vi "Set Timing Source.vi"(8 "error in (no error)":errorcluster, 10 "Timing Source":enum16{"Automatic", "Custom Device"}(ring), 11 "Item Ref in":T1 format="%.0x") -> (0 "error out":errorcluster, 3 "Item Ref out":T1 format="%.0x")   [LabVIEW 2016, in "Scan Engine Custom Device.lvlib"]
uses:
  Scan Engine Custom Device.lvlib
  <vilib>/NI Veristand/Custom Device Tools/Custom Device Utility Library/Custom Device Utility Library.lvlib
  <vilib>/NI Veristand/Custom Device API/Custom Device API.lvlib
  NationalInstruments.VeriStand.SystemStorage
  <vilib>/NI Veristand/Custom Device API/Custom Device Item Ref.ctl
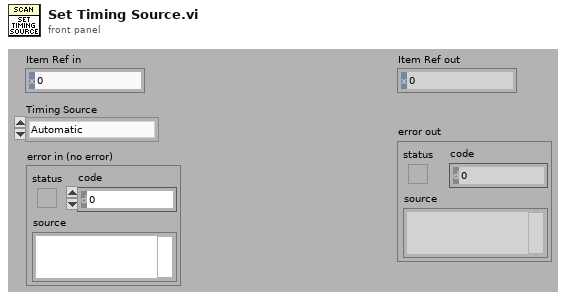
[diagram p1: front panel]
types:
  T1 = typedef "Custom Device API.lvlib/Custom Device Item Ref.ctl" = u64
  T2 = typedef "Custom Device API.lvlib/Custom Device Pointer.ctl" = refnum<k24>
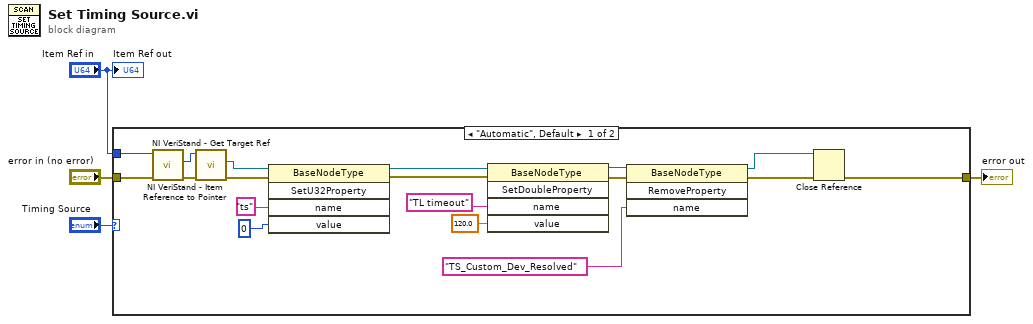
[diagram p0: block diagram]
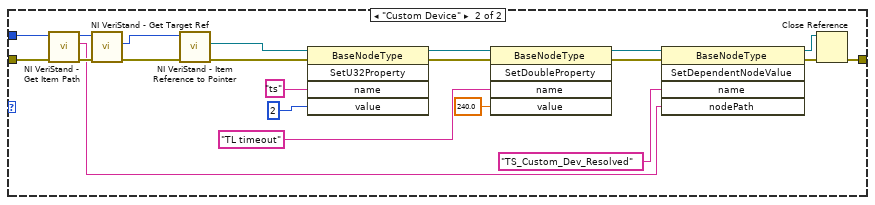
[diagram p2: hidden frame]
diagram:
  n1 = case shown="\"Automatic\", Default" "Timing Source" {
    tunnel: "Item Ref in" -> [w21 w43]
    tunnel: "error in (no error)" -> [w22 w42]
    tunnel: [w11 w29] -> w2
    frame "Automatic", Default {
      n2 = call <vilib>:"NI VeriStand - Get Target Ref.vi"("error in"=w22, "Item Ref in"=w21) -> ("error out"=w20:errorcluster, "Target Ref"=w19:T1)  [unwired: 6 in, 2 out]
      n3 = call <vilib>:"NI VeriStand - Item Reference to Pointer.vi"("error in (no error)"=w20, "Item Ref in"=w19) -> ("error out"=w18:errorcluster, "Node Pointer"=w17:T2)  [unwired: 6 in, 2 out]
      n4 = invoke class="BaseNodeType" method="SetU32Property"(reference=w17, error in=w18, "name"="ts", "value"=u32 0) -> (reference out=w9:T2, error out=w6:errorcluster)  [unwired: 1 in, 3 out]
      n5 = invoke class="BaseNodeType" method="SetDoubleProperty"(reference=w9, error in=w6, "name"="TL timeout", "value"=120.0) -> (reference out=w8:T2, error out=w7:errorcluster)  [unwired: 1 in, 3 out]
      n6 = invoke class="BaseNodeType" method="RemoveProperty"(reference=w8, error in=w7, "name"="TS_Custom_Dev_Resolved") -> (reference out=w13:T2, error out=w12:errorcluster)  [unwired: 1 in, 2 out]
      n7 = Close Reference(reference=w13, error in (no error)=w12) -> (error out=w11:errorcluster)
    }
    frame "Custom Device" {
      n8 = call <vilib>:"NI VeriStand - Get Item Path.vi"("error in (no error)"=w42, "Item Ref in"=w43) -> ("error out"=w41:errorcluster, "Path"=w33:string, "Item Ref out"=w40:T1)  [unwired: 6 in, 1 out]
      n9 = call <vilib>:"NI VeriStand - Get Target Ref.vi"("error in"=w41, "Item Ref in"=w40) -> ("error out"=w39:errorcluster, "Target Ref"=w38:T1)  [unwired: 6 in, 2 out]
      n10 = call <vilib>:"NI VeriStand - Item Reference to Pointer.vi"("error in (no error)"=w39, "Item Ref in"=w38) -> ("error out"=w34:errorcluster, "Node Pointer"=w37:T2)  [unwired: 6 in, 2 out]
      n11 = invoke class="BaseNodeType" method="SetU32Property"(reference=w37, error in=w34, "name"="ts", "value"=u32 2) -> (reference out=w27:T2, error out=w28:errorcluster)  [unwired: 1 in, 3 out]
      n12 = invoke class="BaseNodeType" method="SetDoubleProperty"(reference=w27, error in=w28, "name"="TL timeout", "value"=240.0) -> (reference out=w26:T2, error out=w25:errorcluster)  [unwired: 1 in, 3 out]
      n13 = invoke class="BaseNodeType" method="SetDependentNodeValue"(reference=w26, error in=w25, "name"="TS_Custom_Dev_Resolved", "nodePath"=w33) -> (reference out=w31:T2, error out=w30:errorcluster)  [unwired: 1 in, 3 out]
      n14 = Close Reference(reference=w31, error in (no error)=w30) -> (error out=w29:errorcluster)
    }
  }
  "error out" <- w2
  "Item Ref out" <- "Item Ref in"
